vi "CRYSmoothing Curve.vi"(0 "Data in":T1={"Name"="", "Curve"=[], "X data"=1, "Y data"=1, "Z data"=1, "X axis"=0, "Y axis"=1, "Z axis"=1, "X unit"="Hz", "Y unit"="", "Z unit"="deg.", "X dB ref"=1.0, "Y dB ref"=1.0, "Z dB ref"=1.0, "single val"=FALSE, "protected"=FALSE, "display X"=TRUE, "display Y"=TRUE, "display Z"=TRUE, "Test Info"="", "Step No."=0, "Plot Settings"={"Color"=0, "Interpolation"=0, "Point Style"=0, "Line Style"=0, "Point Color"=0, "Line Width"=0, "Bar Plot Style"=0, "Fill To"=0}, "AutoProtect"=FALSE} {"Z data" items=["dB", "Lin"]; "X data" items=["dB", "Lin"]; "Y data" items=["dB", "Lin"]; "Z dB ref" format="%.1f"; "Z axis" items=["Log", "Lin"]; "X dB ref" format="%.1f"; "X axis" items=["Log", "Lin"]; "Y axis" items=["Log", "Lin"]; "Y dB ref" format="%.1f"; "Curve"."z" format="%.2f"; "Curve"."y" format="%.2f"; "Curve"."x" format="%.2f"}, 5 "Octav Mode":u16(ring) items=["1/1 Octave", "1/3 Octave", "1/6 Octave", "1/12 Octave", "1/24 Octave", "User Defined log", "User Defined lin"], 9 "Octave steps":dbl=1.0 caption="1/n Octave" step=1.0, 11 "Weight Mode":u16(ring) items=["None", "Hanning"]) -> (4 "Resulting data out":T1={"Name"="", "Curve"=[], "X data"=1, "Y data"=1, "Z data"=1, "X axis"=0, "Y axis"=1, "Z axis"=1, "X unit"="Hz", "Y unit"="", "Z unit"="deg.", "X dB ref"=1.0, "Y dB ref"=1.0, "Z dB ref"=1.0, "single val"=FALSE, "protected"=FALSE, "display X"=TRUE, "display Y"=TRUE, "display Z"=TRUE, "Test Info"="", "Step No."=0, "Plot Settings"={"Color"=0, "Interpolation"=0, "Point Style"=0, "Line Style"=0, "Point Color"=0, "Line Width"=0, "Bar Plot Style"=0, "Fill To"=0}, "AutoProtect"=FALSE} {"Z data" items=["dB", "Lin"]; "X data" items=["dB", "Lin"]; "Y data" items=["dB", "Lin"]; "Z dB ref" format="%.1f"; "Z axis" items=["Log", "Lin"]; "X dB ref" format="%.1f"; "X axis" items=["Log", "Lin"]; "Y axis" items=["Log", "Lin"]; "Y dB ref" format="%.1f"; "Curve"."z" format="%.2f"; "Curve"."y" format="%.2f"; "Curve"."x" format="%.2f"}, 10 "error string":string, 15 "Update steps":bool)   [LabVIEW 2013]
uses:
  Typedef Control/CRYData Cluster.ctl
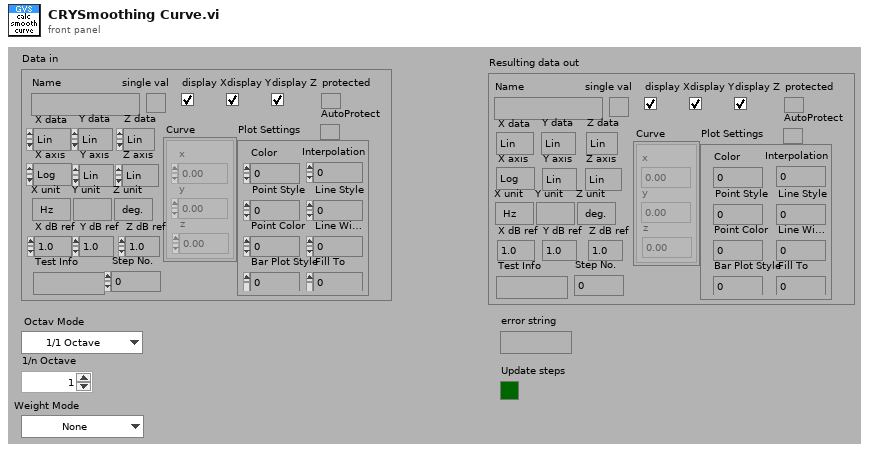
[diagram p1: front panel]
types:
  T1 = typedef "CRYData Cluster.ctl" = cluster{"Name":string, "Curve":cluster{"x":dbl, "y":dbl, "z":dbl}[], "X data":u16, "Y data":u16, "Z data":u16, "X axis":u16, "Y axis":u16, "Z axis":u16, "X unit":string, "Y unit":string, "Z unit":string, "X dB ref":dbl, "Y dB ref":dbl, "Z dB ref":dbl, "single val":bool, "protected":bool, "display X":bool, "display Y":bool, "display Z":bool, "Test Info":string, "Step No.":i32, "Plot Settings":cluster{"Color":u32, "Interpolation":u8, "Point Style":u8, "Line Style":u8, "Point Color":u32, "Line Width":u8, "Bar Plot Style":u8, "Fill To":i16}, "AutoProtect":bool}
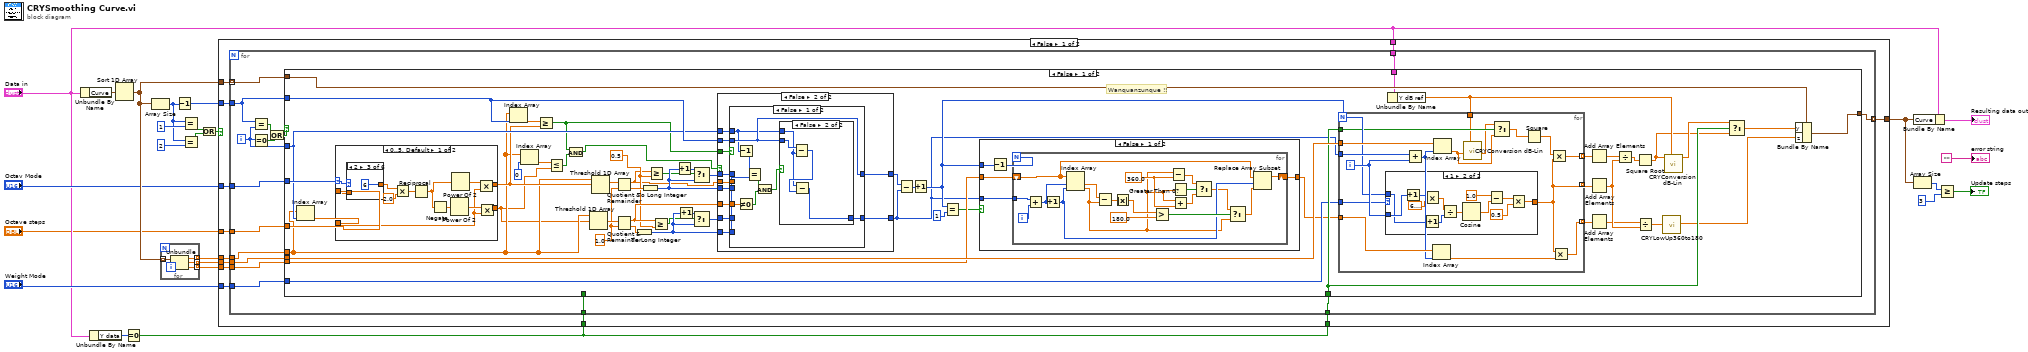
[diagram p0: block diagram]
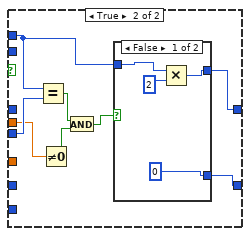
[diagram p4: hidden frame]
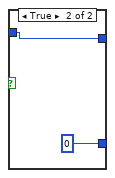
[diagram p5: hidden frame]
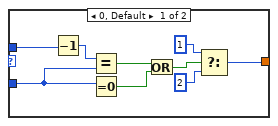
[diagram p6: hidden frame]
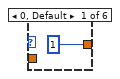
[diagram p7: hidden frame]
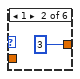
[diagram p8: hidden frame]
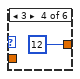
[diagram p9: hidden frame]
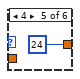
[diagram p10: hidden frame]
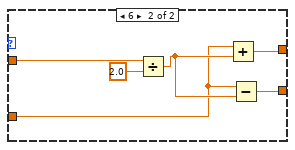
[diagram p12: hidden frame]
diagram:
  n1 = Unbundle By Name("Data in") -> ("Curve"=w16:cluster{"x":dbl, "y":dbl, "z":dbl}[])
  n2 = Unbundle By Name("Data in") -> ("Y data"=w9:u16)
  n3 = Sort 1D Array(array=w16) -> (sorted array=w10:cluster{"x":dbl, "y":dbl, "z":dbl}[])
  n4 = Equal To 0?(x=w9) -> (x = 0?=w1:bool)
  n5 = Array Size(array=w10) -> (size(s)=w21:i32)
  n6 = for {
    tunnel: w10 -> [w28] mode=indexing
    tunnel: [w27] -> w14 mode=indexing
    tunnel: [w26] -> w13 mode=indexing
    tunnel: [w25] -> w15 mode=indexing
    n7 = Unbundle(w28) -> ("x"=w25:dbl, "y"=w27:dbl, "z"=w26:dbl)
  }
  n8 = Decrement(x=w21) -> (x-1=w17:i32)
  n9 = Equal?(x=w21, y=1) -> (x = y?=w19:bool)
  n10 = Equal?(x=w21, y=2) -> (x = y?=w18:bool)
  n11 = Or(x=w19, y=w18) -> (x .or. y?=w11:bool)
  n12 = case shown="False" w11 {
    tunnel: w17 -> [w40 _]
    tunnel: "Octav Mode" -> [w39 _]
    tunnel: w10 -> [w38 w242]
    tunnel: w15 -> [w37 _]
    tunnel: w14 -> [w36 _]
    tunnel: w13 -> [w35 _]
    tunnel: "Weight Mode" -> [w34 _]
    tunnel: "Octave steps" -> [w33 _]
    tunnel: [w32 w242] -> w12
    tunnel: w1 -> [w31 _]
    tunnel: "Data in" -> [w30 _]
    tunnel: w1 -> [w29 _]
    frame False {
      n13 = for {
        tunnel: w38 -> [w53] mode=indexing
        tunnel: w40 -> [w43]
        tunnel: [w52] -> w32 mode=indexing
        tunnel: w39 -> [w51]
        tunnel: w37 -> [w50]
        tunnel: w36 -> [w49]
        tunnel: w35 -> [w48]
        tunnel: w34 -> [w46]
        tunnel: w33 -> [w45]
        tunnel: w31 -> [w44]
        tunnel: w30 -> [w42]
        tunnel: w29 -> [w41]
        i -> [w47]
        n14 = Equal?(x=w43, y=w47) -> (x = y?=w55:bool)
        n15 = Equal To 0?(x=w47) -> (x = 0?=w56:bool)
        n16 = Or(x=w55, y=w56) -> (x .or. y?=w54:bool)
        n17 = case shown="False" w54 {
          tunnel: w53 -> [w111 w241]
          tunnel: [w112 w241] -> w52
          tunnel: w51 -> [w107 _]
          tunnel: w50 -> [w68 _]
          tunnel: w49 -> [w113 _]
          tunnel: w48 -> [w110 _]
          tunnel: w47 -> [w103 _]
          tunnel: w46 -> [w106 _]
          tunnel: w45 -> [w108 _]
          tunnel: w44 -> [w109 _]
          tunnel: w43 -> [w104 _]
          tunnel: w42 -> [w105 _]
          tunnel: w41 -> [_ _]
          frame False {
            w58 = 0.5 ("y")
            w88 = 1.0 ("y")
            # "Wanquanzunque !!"
            n18 = Index Array(array=w68, index=w103) -> (element=w91:dbl)
            n19 = case shown="0..5, Default" w107 {
              selector: w107 -> [w203 _]
              tunnel: w108 -> [w204 w216]
              tunnel: w91 -> [w195 w213]
              tunnel: [w194 w212] -> w76
              tunnel: [w193 w211] -> w66
              frame 0..5, Default {
                n20 = case shown="2" w203 {
                  tunnel: [1 ("y") 3 ("y") 6 ("y") 12 ("y") 24 ("y") w210] -> w202
                  tunnel: w204 -> [_ _ _ _ _ w210]
                  frame 0, Default {
                  }
                  frame 1 {
                  }
                  frame 2 {
                  }
                  frame 3 {
                  }
                  frame 4 {
                  }
                  frame 5 {
                  }
                }
                n21 = Multiply(x=w202, y=2.0) -> (x*y=w200:dbl)
                n22 = Reciprocal(x=w200) -> (1/x=w198:dbl)
                n23 = Negate(x=w198) -> (-x=w199:dbl)
                n24 = Power Of 2(x=w199) -> (2^x=w196:dbl)
                n25 = Power Of 2(x=w198) -> (2^x=w197:dbl)
                n26 = Multiply(x=w197, y=w195) -> (x*y=w194:dbl)
                n27 = Multiply(x=w196, y=w195) -> (x*y=w193:dbl)
              }
              frame 6 {
                n28 = Divide(x=w216, y=2.0) -> (x/y=w214:dbl)
                n29 = Add(x=w213, y=w214) -> (x+y=w212:dbl)
                n30 = Subtract(x=w213, y=w214) -> (x-y=w211:dbl)
              }
            }
            n31 = Index Array(array=w68, index=w104) -> (element=w77:dbl)
            n32 = Index Array(array=w68, index=0) -> (element=w65:dbl)
            n33 = Greater Or Equal?(x=w77, y=w76) -> (x >= y?=w62:bool)
            n34 = Less Or Equal?(x=w65, y=w66) -> (x <= y?=w64:bool)
            n35 = And(x=w62, y=w64) -> (x .and. y?=w63:bool)
            n36 = Threshold 1D Array(2:w66, 3:w68) -> (0:w89:dbl)  [unwired: 1 in]
            n37 = Threshold 1D Array(2:w76, 3:w68) -> (0:w90:dbl)  [unwired: 1 in]
            n38 = Quotient & Remainder(x=w90, y=w88) -> (x-y*floor(x/y)=w57:dbl, floor(x/y)=w87:dbl)
            n39 = Quotient & Remainder(x=w89, y=w88) -> (x-y*floor(x/y)=w60:dbl, floor(x/y)=w84:dbl)
            n40 = To Long Integer(number=w84) -> (32bit integer=w70:i32)
            n41 = To Long Integer(number=w87) -> (32bit integer=w67:i32)
            n42 = Greater Or Equal?(x=w57, y=w58) -> (x >= y?=w59:bool)
            n43 = Greater Or Equal?(x=w60, y=w58) -> (x >= y?=w61:bool)
            n44 = Increment(x=w67) -> (x+1=w86:i32)
            n45 = Increment(x=w70) -> (x+1=w85:i32)
            n46 = Select(t=w86, s=w59, f=w67) -> (s? t:f=w81:i32)
            n47 = Select(t=w85, s=w61, f=w70) -> (s? t:f=w79:i32)
            n48 = case shown="False" w63 {
              tunnel: w104 -> [_ w126]
              tunnel: w103 -> [_ w125]
              tunnel: w81 -> [w115 w124]
              tunnel: [w115 w123] -> w80
              tunnel: w79 -> [w114 w122]
              tunnel: [w114 w121] -> w78
              tunnel: w70 -> [_ w120]
              tunnel: w60 -> [_ w119]
              tunnel: w62 -> [_ w118]
              tunnel: w67 -> [_ w117]
              tunnel: w57 -> [_ w116]
              frame True {
              }
              frame False {
                n49 = case shown="False" w118 {
                  tunnel: w124 -> [_ _]
                  tunnel: [w134 w142] -> w123
                  tunnel: w126 -> [w134 _]
                  tunnel: w122 -> [_ _]
                  tunnel: [w135 w143] -> w121
                  tunnel: w125 -> [w127 w141]
                  tunnel: w120 -> [w132 _]
                  tunnel: w119 -> [w131 _]
                  tunnel: w117 -> [_ w148]
                  tunnel: w116 -> [_ w147]
                  frame False {
                    n50 = Decrement(x=w127) -> (x-1=w133:i32)
                    n51 = Not Equal To 0?(x=w131) -> (x != 0?=w130:bool)
                    n52 = Equal?(x=w133, y=w132) -> (x = y?=w129:bool)
                    n53 = And(x=w129, y=w130) -> (x .and. y?=w128:bool)
                    n54 = case shown="False" w128 {
                      tunnel: [w136 w139] -> w135
                      tunnel: w134 -> [_ w138]
                      tunnel: w127 -> [w136 w137]
                      frame True {
                      }
                      frame False {
                        n55 = Subtract(x=w138, y=w137) -> (x-y=w140:i32)
                        n56 = Subtract(x=w137, y=w140) -> (x-y=w139:i32)
                      }
                    }
                  }
                  frame True {
                    n57 = Equal?(x=w141, y=w148) -> (x = y?=w145:bool)
                    n58 = Not Equal To 0?(x=w147) -> (x != 0?=w144:bool)
                    n59 = And(x=w145, y=w144) -> (x .and. y?=w146:bool)
                    n60 = case shown="False" w146 {
                      tunnel: [0 0] -> w143
                      tunnel: [w149 w153] -> w142
                      tunnel: w141 -> [w150 w153]
                      frame False {
                        n61 = Multiply(x=w150, y=2) -> (x*y=w149:i32)
                      }
                      frame True {
                      }
                    }
                  }
                }
              }
            }
            n62 = Subtract(x=w80, y=w78) -> (x-y=w83:i32)
            n63 = Increment(x=w83) -> (x+1=w82:i32)
            n64 = Equal?(x=w82, y=1) -> (x = y?=w94:bool)
            n65 = case shown="False" w94 {
              tunnel: [w220 w240] -> w96
              tunnel: w110 -> [w219 w240]
              tunnel: w78 -> [w218 _]
              tunnel: w82 -> [w217 _]
              frame False {
                n66 = Decrement(x=w217) -> (x-1=w221:i32)
                n67 = for {
                  N: w221 -> [_]
                  shift-right: [w233] -> w220
                  shift-left: w219 -> [w232]
                  tunnel: w218 -> [w228]
                  i -> [w236]
                  w226 = 360.0 ("x")
                  n68 = Add(x=w228, y=w236) -> (x+y=w229:i32)
                  n69 = Increment(x=w229) -> (x+1=w230:i32)
                  n70 = Index Array(array=w232, index #1=w229, index #2=w230) -> (element #1=w237:dbl, element #2=w225:dbl)
                  n71 = Subtract(x=w237, y=w225) -> (x-y=w238:dbl)
                  n72 = Absolute Value(x=w238) -> (abs(x)=w239:dbl)
                  n73 = Greater?(x=w239, y=180.0) -> (0:w235:bool)
                  n74 = Subtract(x=w225, y=w226) -> (x-y=w224:dbl)
                  n75 = Greater Than 0?(x=w225) -> (x > 0?=w227:bool)
                  n76 = Add(x=w225, y=w226) -> (x+y=w223:dbl)
                  n77 = Select(t=w224, s=w227, f=w223) -> (s? t:f=w222:dbl)
                  n78 = Select(t=w222, s=w235, f=w225) -> (s? t:f=w231:dbl)
                  n79 = Replace Array Subset(array=w232, new element=w231, index=w230) -> (w233:dbl[])
                }
              }
              frame True {
              }
            }
            n80 = Unbundle By Name(w105) -> ("Y dB ref"=w73:dbl)
            n81 = for {
              N: w82 -> [w168]
              tunnel: w78 -> [w171]
              tunnel: w113 -> [w170]
              tunnel: w96 -> [w167]
              tunnel: [w157] -> w102 mode=indexing
              tunnel: [w166] -> w98 mode=indexing
              tunnel: [w165] -> w100 mode=indexing
              tunnel: w109 -> [w162]
              tunnel: w106 -> [w159]
              tunnel: w73 -> [w158]
              i -> [w169]
              n82 = case shown="1" w159 {
                tunnel: w169 -> [w180 w184]
                tunnel: w168 -> [w173 w182]
                tunnel: [w174 w181] -> w157
                frame 0, Default {
                  n83 = Decrement(x=w173) -> (x-1=w172:i32)
                  n84 = Equal?(x=w172, y=w180) -> (x = y?=w179:bool)
                  n85 = Equal To 0?(x=w180) -> (x = 0?=w178:bool)
                  n86 = Or(x=w179, y=w178) -> (x .or. y?=w177:bool)
                  n87 = Select(t=1, s=w177, f=2) -> (s? t:f=w174:i32)
                }
                frame 1 {
                  n88 = Increment(x=w184) -> (x+1=w183:i32)
                  n89 = Increment(x=w182) -> (x+1=w191:i32)
                  n90 = Multiply(x=w183, y=6.283185307179586) -> (x*y=w186:dbl)
                  n91 = Divide(x=w186, y=w191) -> (x/y=w187:dbl)
                  n92 = Cosine(x=w187) -> (cos(x)=w188:dbl)
                  n93 = Subtract(x=1.0, y=w188) -> (x-y=w189:dbl)
                  n94 = Multiply(x=w189, y=0.5) -> (x*y=w181:dbl)
                }
              }
              n95 = Add(x=w171, y=w169) -> (x+y=w164:i32)
              n96 = Index Array(array=w167, index=w164) -> (element=w163:dbl)
              n97 = Index Array(array=w170, index=w164) -> (element=w160:dbl)
              n98 = call "CRYConversion dB-Lin.vi"("dB ref."=w158, "Log In"=w160) -> ("Lin Out"=w161:dbl)  [unwired: 4 in, 3 out]
              n99 = Select(t=w161, s=w162, f=w160) -> (s? t:f=w156:dbl)
              n100 = Square(x=w156) -> (x^2=w155:dbl)
              n101 = Multiply(x=w155, y=w157) -> (x*y=w166:dbl)
              n102 = Multiply(x=w157, y=w163) -> (x*y=w165:dbl)
            }
            n103 = Add Array Elements(numeric array=w98) -> (sum=w97:dbl)
            n104 = Add Array Elements(numeric array=w100) -> (sum=w99:dbl)
            n105 = Add Array Elements(numeric array=w102) -> (sum=w101:dbl)
            n106 = Divide(x=w97, y=w101) -> (x/y=w72:dbl)
            n107 = Square Root(x=w72) -> (sqrt(x)=w71:dbl)
            n108 = Divide(x=w99, y=w101) -> (x/y=w75:dbl)
            n109 = call "CRYLowUp360to180.vi"("Value In"=w75) -> ("Value Out"=w74:dbl)  [unwired: 10 in]
            n110 = call "CRYConversion dB-Lin.vi"("dB ref."=w73, "Lin In"=w71) -> ("Log Out"=w93:dbl)  [unwired: 4 in, 3 out]
            n111 = Select(t=w93, s=w109, f=w71) -> (s? t:f=w92:dbl)
            n112 = Bundle By Name(cluster=w111, "y"=w92, "z"=w74) -> (w112:cluster{"x":dbl, "y":dbl, "z":dbl})
          }
          frame True {
          }
        }
      }
    }
    frame True {
    }
  }
  n113 = Bundle By Name(cluster="Data in", "Curve"=w12) -> (→"Resulting data out":T1)
  n114 = Array Size(array=w12) -> (size(s)=w24:i32)
  n115 = Greater Or Equal?(x=w24, y=3) -> (x >= y?=→"Update steps":bool)
  "error string" <- ""
